vi "Autonomous Independent.vi"() -> ()   [LabVIEW 2011]
doc: "This VI is called when autonomous begins, and will automatically be terminated when autonomous ends. You can carry out timed or sensor driven robot movement independently without needing to return to the caller."
uses:
  Robot Global Data.vi
panel:
  in  "DWFNBL":u16=350
  in  "DWFNBH":u16=350
  in  "SWFHBM":dbl=0.27
  in  "SWFMBM":dbl
  in  "SWFLBM":dbl
  in  "Time":dbl=21.6
  in  "Distance wanted for neutral bridge":u16=350
  in  "SWFHB":dbl=963.13
  in  "SWFMB":dbl=700.0
  in  "SWFLB":dbl
  in  "DWFMB":u16
  in  "DWFLB":u16
  in  "DistanceWanted":u16
  in  "WhereAmI":T1(ring)
  in  "NumOfBalls":u8
  in  "Delay":dbl
  in  "DriveToBridgeInstantly?":bool
  in  "DriveToBridge?":bool
  in  "State":T2(ring)
  # "Shotting speed"
  # "By Encoder"
  # "By Battery%"
  # "High"
  # "Middle"
  # "Low"
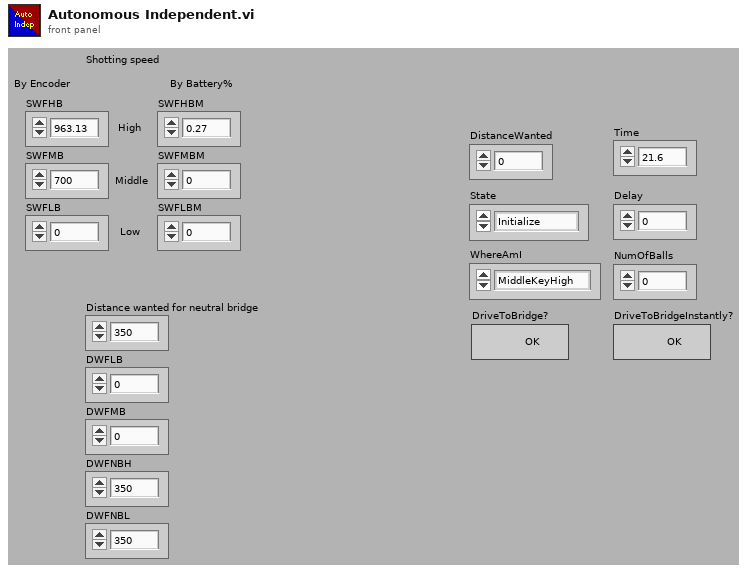
[diagram p1: front panel]
types:
  T1 = enum16{"MiddleKeyHigh", "MiddleKeyLow", "SidesKey"}
  T2 = enum16{"Initialize", "Delay", "Drive", "GetSpeed", "Shoot", "Spin", "DriveToBridge", "Finish"}
  T3 = typedef "WPI_EncoderDevRef.ctl" = cluster{"DevStatus":errorcluster, "EncoderIndex":T4, "CounterIndex":T5, "DistancePerCount":dbl, "Decoding Type":T6}
  T4 = typedef "FPGA_EncoderIdx.ctl" = enum8{"Enc 0", "Enc 1", "Enc 2", "Enc 3", "Invalid"}
  T5 = typedef "FPGA_CounterCtrSystemIndex.ctl" = enum8{"Ctr 0", "Ctr 1", "Ctr 2", "Ctr 3", "Ctr 4", "Ctr 5", "Ctr 6", "Ctr 7", "Invalid"}
  T6 = typedef "WPI_EncoderType.ctl" = enum16{"1x", "2x", "4x"}
  T7 = typedef "WPI_GyroDevRef.ctl" = cluster{"DevStatus":errorcluster, "Analog Module":T8, "Analog Channel":T9, "Offset":dbl, "Gain (VoltsPerDegree/Second)":dbl}
  T8 = typedef "FPGA_TypedefAnalogModule.ctl" = enum16{"Analog Module 1", "Analog Module 2"}
  T9 = typedef "FPGA_AIChannel.ctl" = enum8{"AI 1", "AI 2", "AI 3", "AI 4", "AI 5", "AI 6", "AI 7", "AI 8", "Invalid"}
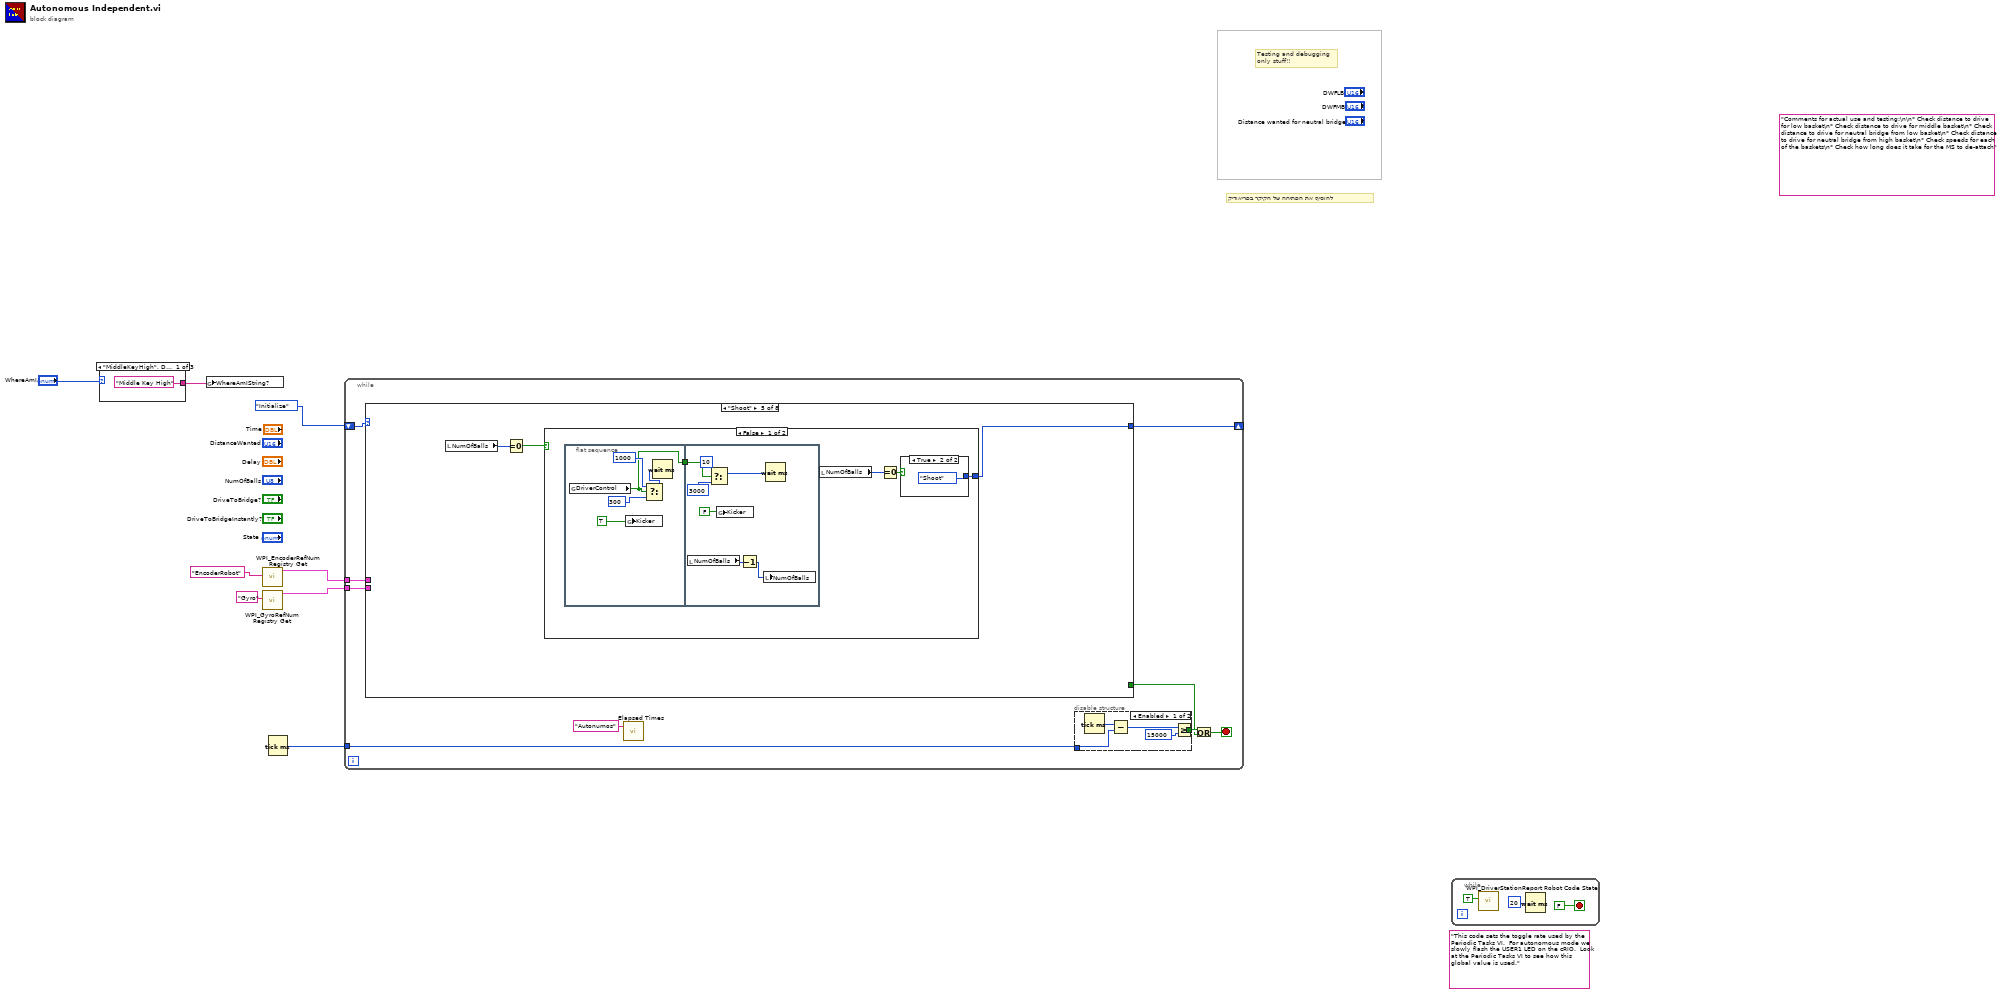
[diagram p0: block diagram]
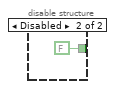
[diagram p2: hidden frame]
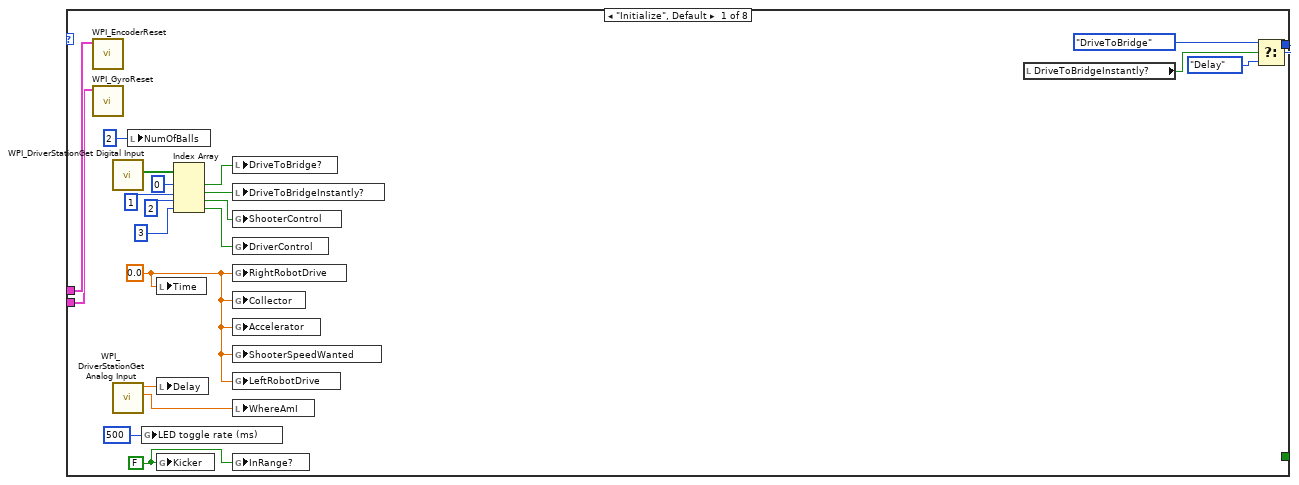
[diagram p3: hidden frame]
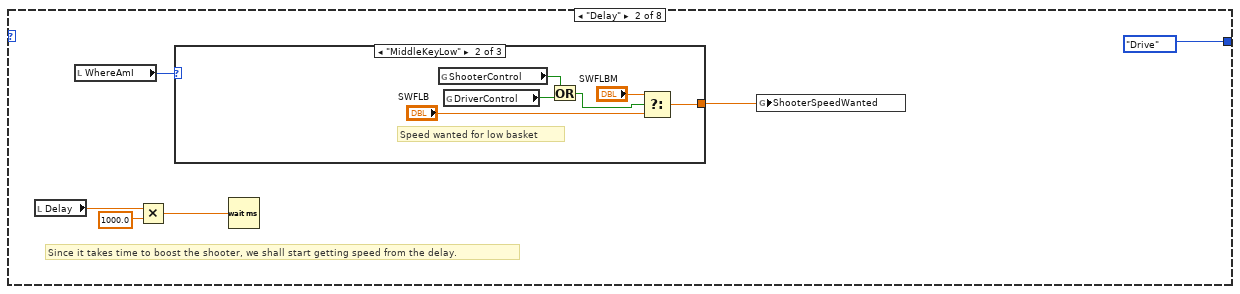
[diagram p4: hidden frame]
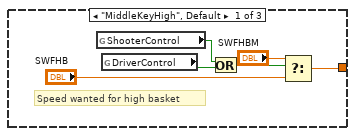
[diagram p5: hidden frame]
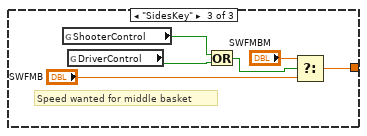
[diagram p6: hidden frame]
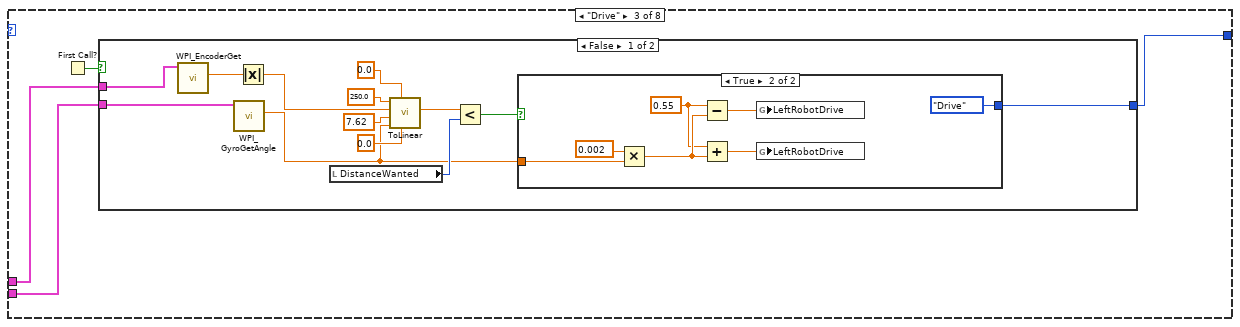
[diagram p7: hidden frame]
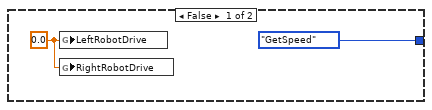
[diagram p8: hidden frame]
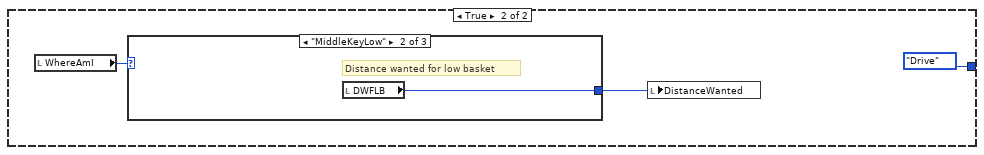
[diagram p9: hidden frame]
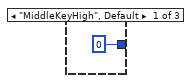
[diagram p10: hidden frame]
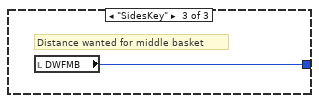
[diagram p11: hidden frame]
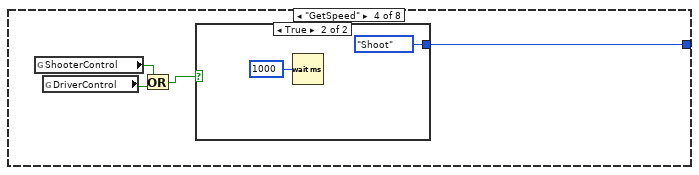
[diagram p12: hidden frame]
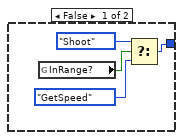
[diagram p13: hidden frame]
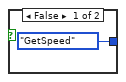
[diagram p14: hidden frame]
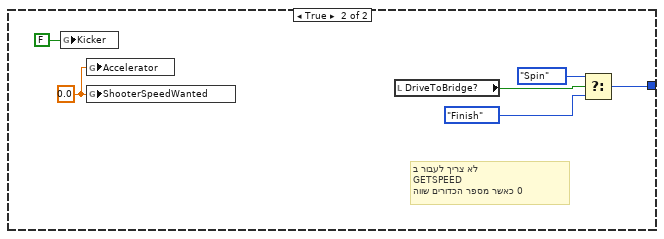
[diagram p15: hidden frame]
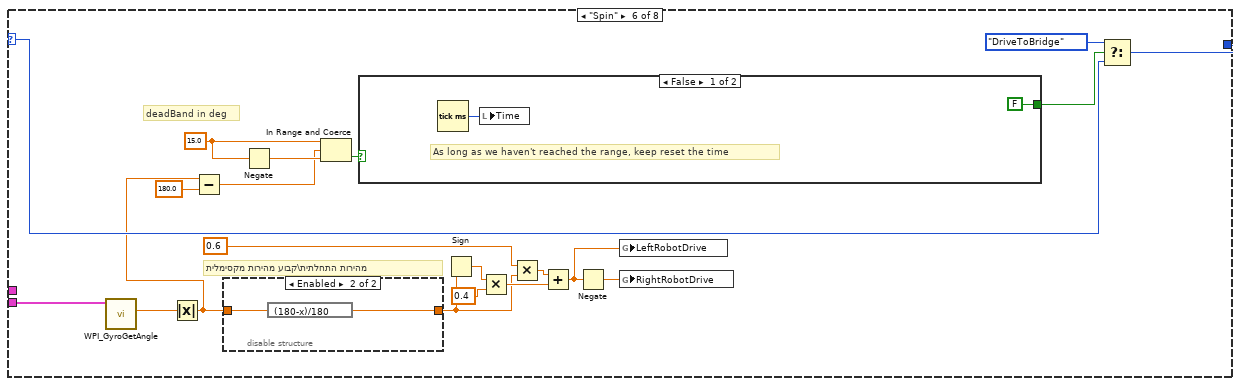
[diagram p16: hidden frame]
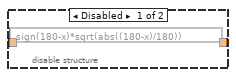
[diagram p17: hidden frame]
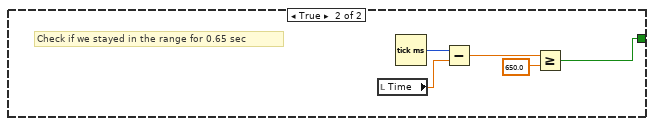
[diagram p18: hidden frame]
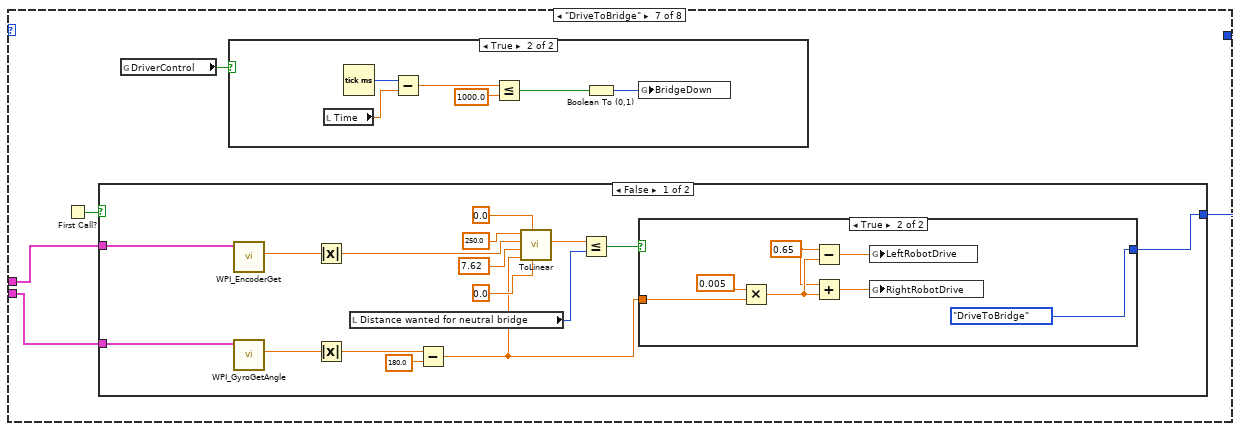
[diagram p19: hidden frame]
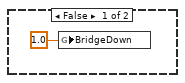
[diagram p20: hidden frame]
diagram:
  (unwired) "Comments for actual use and testing:\n\n* Check distance to drive for low basket\n* Check distance to drive for middle basket\n* Check distance to drive for neutral bridge from low basket\n* Check distance to drive for neutral bridge from high basket\n* Check speeds for each of the baskets\n* Check how long does it take for the MS to de-attach"
  (unwired) "This code sets the toggle rate used by the Periodic Tasks VI.  For autonomous mode we slowly flash the USER1 LED on the cRIO.  Look at the Periodic Tasks VI to see how this global value is used."
  # "להוסיף את הפתיחה של הקיקר בפריאודיק"
  # "Testing and debugging\nonly stuff!!"
  n1 = case shown="\"MiddleKeyHigh\", Default" "WhereAmI" {
    tunnel: ["Middle Key High" "Middle Key Low" "Sides Key"] -> w1
    frame "MiddleKeyHigh", Default {
    }
    frame "MiddleKeyLow" {
    }
    frame "SidesKey" {
    }
  }
  n2 = global write "Robot Global Data.vi" "WhereAmIString?"(w1) -> ()
  n3 = call <vilib>:"WPI_EncoderRefNum Registry Get.vi"("refnum name"="EncoderRobot") -> ("EncoderDevRef"=w7:T3)  [unwired: 9 in, 1 out]
  n4 = call <vilib>:"WPI_GyroRefNum Registry Get.vi"("refnum name"="Gyro") -> ("GyroDevRef"=w6:T7)  [unwired: 9 in, 1 out]
  n5 = Tick Count (ms)() -> (millisecond timer value=w4:u32)
  n6 = while {
    shift-right: [w18] -> _
    shift-left: T2."Initialize" ("State") -> [w14]
    tunnel: w7 -> [w20]
    tunnel: w6 -> [w19]
    tunnel: w4 -> [w17]
    stop <- w15 stop-if-true
    n7 = case shown="\"Shoot\"" w14 {
      selector: w14 -> [_ _ _ _ _ w157 _ _]
      tunnel: w20 -> [w40 _ w72 _ _ _ w175 _]
      tunnel: w19 -> [w39 _ w74 _ _ w160 w174 _]
      tunnel: [w35 T2."Drive" ("State") w73 w107 w114 w156 w173 T2."Finish" ("State")] -> w18
      tunnel: [_ _ _ _ _ _ _ TRUE] -> w12
      frame "Initialize", Default {
        w37 = 0.0
        w38 = FALSE
        n8 = call <vilib>:"WPI_EncoderReset.vi"("EncoderDevRef"=w40) -> ()  [unwired: 9 in, 2 out]
        n9 = call <vilib>:"WPI_GyroReset.vi"("GyroDevRef"=w39) -> ()  [unwired: 9 in, 2 out]
        n10 = call <vilib>:"WPI_DriverStationGet Digital Input.vi"() -> ("Driver Station Digital Input (1-8)"=w45:bool[])  [unwired: 11 in]
        n11 = call <vilib>:"WPI_DriverStationGet Analog Input.vi"() -> ("Analog 2 (V)"=w46:dbl, "Analog 1 (V)"=w47:dbl)  [unwired: 8 in, 2 out]
        n12 = local write "NumOfBalls"(u8 2 ("NumOfBalls")) -> ()
        n13 = global write "Robot Global Data.vi" "LED toggle rate (ms)"(u32 500 ("LED ms toggle rate")) -> ()
        n14 = local write "Time"(w37) -> ()
        n15 = local write "Delay"(w47) -> ()
        n16 = global write "Robot Global Data.vi" "Kicker"(w38) -> ()
        n17 = Index Array(array=w45, index #1=0 ("index"), index #2=1 ("index"), index #3=2 ("index"), index #4=3 ("index")) -> (element #1=w44:bool, element #2=w43:bool, element #3=w32:bool, element #4=w31:bool)
        n18 = local write "DriveToBridge?"(w44) -> ()
        n19 = local write "DriveToBridgeInstantly?"(w43) -> ()
        n20 = global write "Robot Global Data.vi" "ShooterControl"(w32) -> ()
        n21 = global write "Robot Global Data.vi" "DriverControl"(w31) -> ()
        n22 = global write "Robot Global Data.vi" "RightRobotDrive"(w37) -> ()
        n23 = global write "Robot Global Data.vi" "Collector"(w37) -> ()
        n24 = global write "Robot Global Data.vi" "Accelerator"(w37) -> ()
        n25 = global write "Robot Global Data.vi" "ShooterSpeedWanted"(w37) -> ()
        n26 = global write "Robot Global Data.vi" "LeftRobotDrive"(w37) -> ()
        n27 = local write "WhereAmI"(w46) -> ()
        n28 = global write "Robot Global Data.vi" "InRange?"(w38) -> ()
        n29 = local read "DriveToBridgeInstantly?"() -> (w36:bool)
        n30 = Select(t=T2."DriveToBridge" ("State"), s=w36, f=T2."Delay" ("State")) -> (s? t:f=w35:T2)
      }
      frame "Delay" {
        # "Since it takes time to boost the shooter, we shall start getting speed from the delay."
        n31 = local read "Delay"() -> (w53:dbl)
        n32 = local read "WhereAmI"() -> (w50:T1)
        n33 = Multiply(x=w53, y=1000.0) -> (x*y=w51:dbl)
        n34 = case shown="\"MiddleKeyLow\"" w50 {
          tunnel: [w59 w65 w71] -> w49
          frame "MiddleKeyHigh", Default {
            # "Speed wanted for high basket"
            n35 = global read "Robot Global Data.vi" "ShooterControl"() -> (w56:bool)
            n36 = global read "Robot Global Data.vi" "DriverControl"() -> (w55:bool)
            n37 = Or(x=w56, y=w55) -> (x .or. y?=w54:bool)
            n38 = Select(t="SWFHBM", s=w54, f="SWFHB") -> (s? t:f=w59:dbl)
          }
          frame "MiddleKeyLow" {
            # "Speed wanted for low basket"
            n39 = global read "Robot Global Data.vi" "ShooterControl"() -> (w62:bool)
            n40 = global read "Robot Global Data.vi" "DriverControl"() -> (w61:bool)
            n41 = Or(x=w62, y=w61) -> (x .or. y?=w60:bool)
            n42 = Select(t="SWFLBM", s=w60, f="SWFLB") -> (s? t:f=w65:dbl)
          }
          frame "SidesKey" {
            # "Speed wanted for middle basket"
            n43 = global read "Robot Global Data.vi" "ShooterControl"() -> (w68:bool)
            n44 = global read "Robot Global Data.vi" "DriverControl"() -> (w67:bool)
            n45 = Or(x=w68, y=w67) -> (x .or. y?=w66:bool)
            n46 = Select(t="SWFMBM", s=w66, f="SWFMB") -> (s? t:f=w71:dbl)
          }
        }
        n47 = Wait (ms)(milliseconds to wait=w51) -> ()  [unwired: 1 out]
        n48 = global write "Robot Global Data.vi" "ShooterSpeedWanted"(w49) -> ()
      }
      frame "Drive" {
        n49 = First Call?() -> (First Call?: T/F=w75:bool)
        n50 = case shown="False" w75 {
          tunnel: w74 -> [w86 _]
          tunnel: [w76 T2."Drive" ("State")] -> w73
          tunnel: w72 -> [w77 _]
          frame False {
            n51 = call <vilib>:"WPI_EncoderGet.vi"("EncoderDevRef"=w77) -> ("Distance"=w88:dbl)  [unwired: 5 in, 5 out]
            n52 = call <vilib>:"WPI_GyroGetAngle.vi"("GyroDevRef"=w86) -> ("Angle"=w78:dbl)  [unwired: 7 in, 3 out]
            n53 = Absolute Value(x=w88) -> (abs(x)=w87:dbl)
            n54 = local read "DistanceWanted"() -> (w79:u16)
            n55 = call "ToLinear.vi"("NumberOfTicks"=0.0, "DistanceTraveled"=0.0, "Angle"=w78, "R"=7.62, "EncoderRate"=w87, "EncoderTicks"=250.0) -> ("DistanceTraveledO"=w81:dbl)  [unwired: 3 in]
            n56 = Less?(x=w81, y=w79) -> (x < y?=w80:bool)
            n57 = case shown="True" w80 {
              tunnel: [T2."GetSpeed" ("State") T2."Drive" ("State")] -> w76
              tunnel: w78 -> [_ w96]
              frame False {
                w90 = 0.0 ("MotorDriveLeft")
                n58 = global write "Robot Global Data.vi" "LeftRobotDrive"(w90) -> ()
                n59 = global write "Robot Global Data.vi" "RightRobotDrive"(w90) -> ()
              }
              frame True {
                w94 = 0.55
                n60 = Multiply(x=0.002, y=w96) -> (x*y=w95:dbl)
                n61 = Subtract(x=w94, y=w95) -> (x-y=w93:dbl)
                n62 = Add(x=w94, y=w95) -> (x+y=w92:dbl)
                n63 = global write "Robot Global Data.vi" "LeftRobotDrive"(w93) -> ()
                n64 = global write "Robot Global Data.vi" "LeftRobotDrive"(w92) -> ()
              }
            }
          }
          frame True {
            n65 = local read "WhereAmI"() -> (w100:T1)
            n66 = case shown="\"MiddleKeyLow\"" w100 {
              tunnel: [u16 0 ("Distance wanted for middle basket") w102 w103] -> w99
              frame "MiddleKeyHigh", Default {
              }
              frame "MiddleKeyLow" {
                # "Distance wanted for low basket"
                n67 = local read "DWFLB"() -> (w102:u16)
              }
              frame "SidesKey" {
                # "Distance wanted for middle basket"
                n68 = local read "DWFMB"() -> (w103:u16)
              }
            }
            n69 = local write "DistanceWanted"(w99) -> ()
          }
        }
      }
      frame "GetSpeed" {
        n70 = global read "Robot Global Data.vi" "ShooterControl"() -> (w106:bool)
        n71 = global read "Robot Global Data.vi" "DriverControl"() -> (w105:bool)
        n72 = Or(x=w106, y=w105) -> (x .or. y?=w104:bool)
        n73 = case shown="True" w104 {
          tunnel: [w108 T2."Shoot" ("State")] -> w107
          frame False {
            n74 = global read "Robot Global Data.vi" "InRange?"() -> (w111:bool)
            n75 = Select(t=T2."Shoot" ("State"), s=w111, f=T2."GetSpeed" ("State")) -> (s? t:f=w108:T2)
          }
          frame True {
            n76 = Wait (ms)(milliseconds to wait=u32 1000) -> ()  [unwired: 1 out]
          }
        }
      }
      frame "Shoot" {
        n77 = local read "NumOfBalls"() -> (w115:u8)
        n78 = Equal To 0?(x=w115) -> (x = 0?=w116:bool)
        n79 = case shown="False" w116 {
          tunnel: [w120 w137] -> w114
          frame False {
            n80 = flat-sequence {
              tunnel: [w123] -> w118
              tunnel: w118 -> [w131]
              frame #0 {
                n81 = global read "Robot Global Data.vi" "DriverControl"() -> (w123:bool)
                n82 = global write "Robot Global Data.vi" "Kicker"(TRUE ("ButtonKicker")) -> ()
                n83 = Select(t=u32 1000 ("f"), s=w123, f=u32 300 ("milliseconds to wait")) -> (s? t:f=w126:u32)
                n84 = Wait (ms)(milliseconds to wait=w126) -> ()  [unwired: 1 out]
              }
              frame #1 {
                n85 = local read "NumOfBalls"() -> (w133:u8)
                n86 = Select(t=u32 10, s=w131, f=u32 3000 ("milliseconds to wait")) -> (s? t:f=w129:u32)
                n87 = global write "Robot Global Data.vi" "Kicker"(FALSE ("ButtonKicker")) -> ()
                n88 = Decrement(x=w133) -> (x-1=w132:u8)
                n89 = local write "NumOfBalls"(w132) -> ()
                n90 = Wait (ms)(milliseconds to wait=w129) -> ()  [unwired: 1 out]
              }
            }
            n91 = local read "NumOfBalls"() -> (w119:u8)
            n92 = Equal To 0?(x=w119) -> (x = 0?=w117:bool)
            n93 = case shown="True" w117 {
              tunnel: [T2."GetSpeed" ("State") T2."Shoot" ("State")] -> w120
              frame False {
              }
              frame True {
              }
            }
          }
          frame True {
            w139 = 0.0 ("Accelerator")
            # "לא צריך לעבור ב\nGETSPEED\nכאשר מספר הכדורים שווה 0"
            n94 = global write "Robot Global Data.vi" "Kicker"(FALSE ("ButtonKicker")) -> ()
            n95 = global write "Robot Global Data.vi" "Accelerator"(w139) -> ()
            n96 = global write "Robot Global Data.vi" "ShooterSpeedWanted"(w139) -> ()
            n97 = local read "DriveToBridge?"() -> (w140:bool)
            n98 = Select(t=T2."Spin" ("State"), s=w140, f=T2."Finish" ("State")) -> (s? t:f=w137:T2)
          }
        }
      }
      frame "Spin" {
        w153 = 15.0 ("upper limit")
        # "deadBand in deg"
        # "קבוע מהירות מקסימלית\\מהירות התחלתית"
        n99 = call <vilib>:"WPI_GyroGetAngle.vi"("GyroDevRef"=w160) -> ("Angle"=w158:dbl)  [unwired: 7 in, 3 out]
        n100 = Absolute Value(x=w158) -> (abs(x)=w143:dbl)
        n101 = Subtract(x=w143, y=180.0) -> (x-y=w142:dbl)
        n102 = disable-structure shown="Enabled" {
          disable-tunnel: [w162 w164] -> w146
          disable-tunnel: w143 -> [w161 w163]
          frame Disabled {
            n103 = expression code="sign(180-x)*sqrt(abs((180-x)/180))"(w161) -> (w162:dbl)
          }
          frame Enabled {
            n104 = expression code="(180-x)/180"(w163) -> (w164:dbl)
          }
        }
        n105 = Negate(x=w153) -> (-x=w154:dbl)
        n106 = In Range and Coerce(upper limit=w153, x=w142, lower limit=w154) -> (In Range?=w152:bool)  [unwired: 1 out]
        n107 = case shown="False" w152 {
          tunnel: [FALSE w167] -> w151
          frame False {
            # "As long as we haven't reached the range, keep reset the time"
            n108 = Tick Count (ms)() -> (millisecond timer value=w166:u32)
            n109 = local write "Time"(w166) -> ()
          }
          frame True {
            # "Check if we stayed in the range for 0.65 sec"
            n110 = local read "Time"() -> (w170:dbl)
            n111 = Tick Count (ms)() -> (millisecond timer value=w169:u32)
            n112 = Subtract(x=w169, y=w170) -> (x-y=w171:dbl)
            n113 = Greater Or Equal?(x=w171, y=650.0) -> (x >= y?=w167:bool)
          }
        }
        n114 = Sign(1:w146) -> (0:w141:dbl)
        n115 = Multiply(x=w141, y=0.4) -> (x*y=w147:dbl)
        n116 = Multiply(x=0.6, y=w146) -> (x*y=w148:dbl)
        n117 = Add(x=w148, y=w147) -> (x+y=w149:dbl)
        n118 = Negate(x=w149) -> (-x=w150:dbl)
        n119 = global write "Robot Global Data.vi" "LeftRobotDrive"(w149) -> ()
        n120 = global write "Robot Global Data.vi" "RightRobotDrive"(w150) -> ()
        n121 = Select(t=T2."DriveToBridge" ("State"), s=w151, f=w157) -> (s? t:f=w156:T2)
      }
      frame "DriveToBridge" {
        n122 = First Call?() -> (First Call?: T/F=w176:bool)
        n123 = case shown="False" w176 {
          tunnel: w175 -> [w187 w213]
          tunnel: w174 -> [w186 _]
          tunnel: [w185 T2."DriveToBridge" ("State")] -> w173
          frame False {
            n124 = call <vilib>:"WPI_EncoderGet.vi"("EncoderDevRef"=w187) -> ("Distance"=w184:dbl)  [unwired: 5 in, 5 out]
            n125 = call <vilib>:"WPI_GyroGetAngle.vi"("GyroDevRef"=w186) -> ("Angle"=w191:dbl)  [unwired: 7 in, 3 out]
            n126 = Absolute Value(x=w184) -> (abs(x)=w199:dbl)
            n127 = Absolute Value(x=w191) -> (abs(x)=w188:dbl)
            n128 = local read "Distance wanted for neutral bridge"() -> (w192:u16)
            n129 = Subtract(x=w188, y=180.0) -> (x-y=w190:dbl)
            n130 = call "ToLinear.vi"("NumberOfTicks"=0.0, "DistanceTraveled"=0.0, "Angle"=w190, "R"=7.62, "EncoderRate"=w199, "EncoderTicks"=250.0) -> ("DistanceTraveledO"=w194:dbl)  [unwired: 3 in]
            n131 = Less Or Equal?(x=w194, y=w192) -> (x <= y?=w193:bool)
            n132 = case shown="True" w193 {
              tunnel: [T2."Finish" ("State") T2."DriveToBridge" ("State")] -> w185
              tunnel: w190 -> [_ w205]
              frame False {
                w201 = 0.0 ("MotorDriveLeft")
                n133 = global write "Robot Global Data.vi" "RightRobotDrive"(w201) -> ()
                n134 = global write "Robot Global Data.vi" "LeftRobotDrive"(w201) -> ()
              }
              frame True {
                w203 = 0.65
                n135 = Multiply(x=0.005, y=w205) -> (x*y=w204:dbl)
                n136 = Subtract(x=w203, y=w204) -> (x-y=w207:dbl)
                n137 = Add(x=w203, y=w204) -> (x+y=w206:dbl)
                n138 = global write "Robot Global Data.vi" "LeftRobotDrive"(w207) -> ()
                n139 = global write "Robot Global Data.vi" "RightRobotDrive"(w206) -> ()
              }
            }
          }
          frame True {
            w214 = 0.0
            n140 = call <vilib>:"WPI_EncoderReset.vi"("EncoderDevRef"=w213) -> ()  [unwired: 9 in, 2 out]
            n141 = Tick Count (ms)() -> (millisecond timer value=w209:u32)
            n142 = local read "WhereAmI"() -> (w212:T1)
            n143 = global write "Robot Global Data.vi" "LeftRobotDrive"(w214) -> ()
            n144 = global write "Robot Global Data.vi" "RightRobotDrive"(w214) -> ()
            n145 = local write "Time"(w209) -> ()
            n146 = case shown="\"SidesKey\"" w212 {
              tunnel: ["DWFNBL" "DWFNBH" u16 0 ("DWFNBH")] -> w211
              frame "MiddleKeyLow" {
              }
              frame "MiddleKeyHigh" {
              }
              frame "SidesKey" {
              }
            }
            n147 = local write "Distance wanted for neutral bridge"(w211) -> ()
          }
        }
        n148 = global read "Robot Global Data.vi" "DriverControl"() -> (w172:bool)
        n149 = case shown="True" w172 {
          frame False {
            n150 = global write "Robot Global Data.vi" "BridgeDown"(1.0 ("BridgeDown")) -> ()
          }
          frame True {
            n151 = local read "Time"() -> (w182:dbl)
            n152 = Tick Count (ms)() -> (millisecond timer value=w183:u32)
            n153 = Subtract(x=w183, y=w182) -> (x-y=w181:dbl)
            n154 = Less Or Equal?(x=w181, y=1000.0) -> (x <= y?=w179:bool)
            n155 = Boolean To (0,1)(Boolean=w179) -> (0, 1=w178:i16)
            n156 = global write "Robot Global Data.vi" "BridgeDown"(w178) -> ()
          }
        }
      }
      frame "Finish" {
        w221 = 0.0
        w222 = FALSE
        n157 = global write "Robot Global Data.vi" "DriverControl"(FALSE ("DriverControl")) -> ()
        n158 = global write "Robot Global Data.vi" "Kicker"(w222) -> ()
        n159 = local write "Time"(w221) -> ()
        n160 = global write "Robot Global Data.vi" "InRange?"(w222) -> ()
        n161 = global write "Robot Global Data.vi" "RightRobotDrive"(w221) -> ()
        n162 = global write "Robot Global Data.vi" "Collector"(w221) -> ()
        n163 = global write "Robot Global Data.vi" "Accelerator"(w221) -> ()
        n164 = global write "Robot Global Data.vi" "ShooterSpeedWanted"(w221) -> ()
        n165 = global write "Robot Global Data.vi" "LeftRobotDrive"(w221) -> ()
      }
    }
    n166 = call "Elapsed Times.vi"("Call Name"="Autonumos") -> ()  [unwired: 2 in, 1 out]
    n167 = disable-structure shown="Enabled" {
      disable-tunnel: w17 -> [w22 _]
      disable-tunnel: [w21 FALSE] -> w16
      frame Enabled {
        n168 = Tick Count (ms)() -> (millisecond timer value=w25:u32)
        n169 = Subtract(x=w25, y=w22) -> (x-y=w24:u32)
        n170 = Greater Or Equal?(x=w24, y=u32 15000) -> (x >= y?=w21:bool)
      }
      frame Disabled {
      }
    }
    n171 = Or(x=w16, y=w12) -> (x .or. y?=w15:bool)
  }
  n172 = while {
    stop <- FALSE stop-if-true
    n173 = call <vilib>:"WPI_DriverStationReport Robot Code State.vi"("Autonomous"=TRUE) -> ()  [unwired: 10 in, 1 out]
    n174 = Wait (ms)(milliseconds to wait=u32 20) -> ()  [unwired: 1 out]
  }
